vi "grade.vi"(5 "A":dbl format="%#_13g", 9 "S":dbl format="%#_13g") -> (8 "V":dbl)   [LabVIEW 2019]
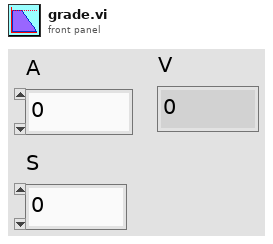
[diagram p1: front panel]
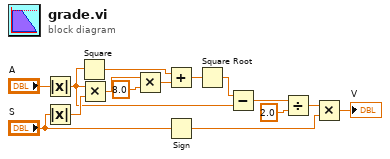
[diagram p0: block diagram]
diagram:
  n1 = Absolute Value(x="A") -> (abs(x)=w7:dbl)
  n2 = Absolute Value(x="S") -> (abs(x)=w13:dbl)
  n3 = Square(x=w7) -> (x^2=w14:dbl)
  n4 = Multiply(x=w7, y=w13) -> (x*y=w12:dbl)
  n5 = Multiply(x=w12, y=8.0) -> (x*y=w10:dbl)
  n6 = Add(x=w14, y=w10) -> (x+y=w9:dbl)
  n7 = Sign(1:"S") -> (0:w1:dbl)
  n8 = Square Root(x=w9) -> (sqrt(x)=w8:dbl)
  n9 = Subtract(x=w8, y=w7) -> (x-y=w6:dbl)
  n10 = Divide(x=w6, y=2.0) -> (x/y=w4:dbl)
  n11 = Multiply(x=w4, y=w1) -> (x*y=→"V":dbl)
